vi "Create One Timeset.vi"(6 "timeset name":string="-", 7 "Notes":string, 8 "error in (no error)":errorcluster, 9 "Pin State":T1[](array[typedef]), 10 "opcode":string, 11 "BML Pattern Creater in":refnum<class "BML Pattern Creater.lvclass">) -> (0 "error out":errorcluster, 2 "string out":string, 3 "BML Pattern Creater out":refnum<class "BML Pattern Creater.lvclass">)   [LabVIEW 2018, in "BML Pattern Creater.lvlib" / "BML Pattern Creater.lvclass"]
uses:
  BML Pattern Creater.lvclass
  Interfaces/Protocol Interface.lvlibp/Interfaces/Protocol Interface/Pin State.ctl
  Interfaces/Protocol Interface.lvlibp/Interfaces/Protocol Interface/Protocol Interface.lvclass
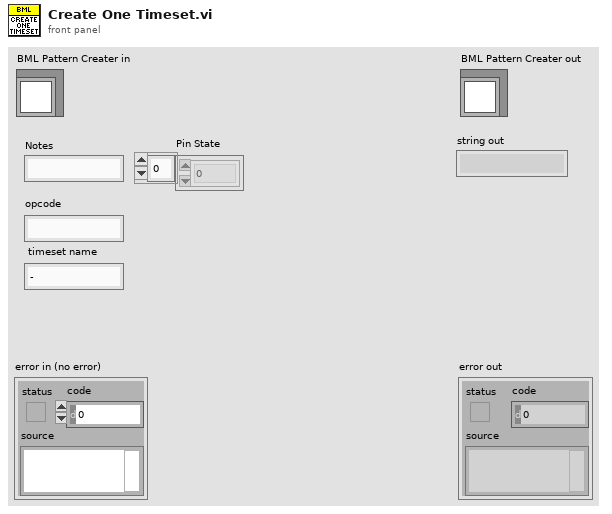
[diagram p1: front panel]
types:
  T1 = typedef "Protocol Interface.lvlibp/Protocol Interface.lvclass/Pin State.ctl" = enum16{"0", "1", "L", "H", "X", "V", "D", "M"}
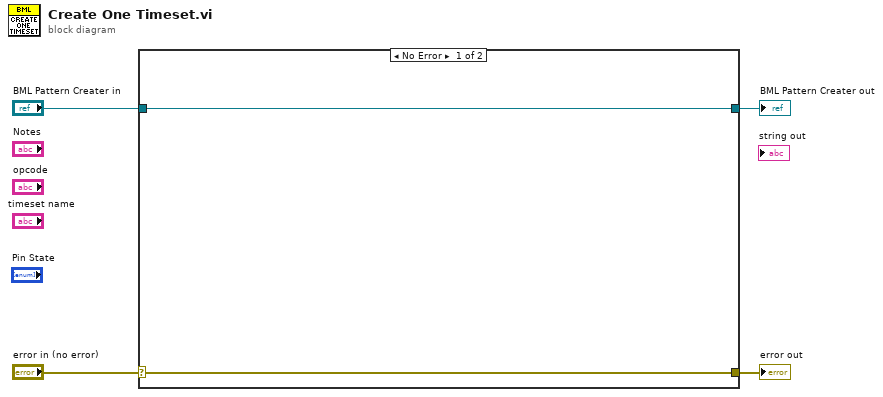
[diagram p0: block diagram]
diagram:
  n1 = case shown="No Error" "error in (no error)" {
    selector: "error in (no error)" -> [w5 w8]
    tunnel: [w5 w8] -> w3
    tunnel: [w6 w7] -> w1
    tunnel: "BML Pattern Creater in" -> [w6 w7]
    frame No Error {
    }
    frame Error {
    }
  }
  "error out" <- w3
  "BML Pattern Creater out" <- w1
